vi "Write Cell T2.vi"(8 "error in (no error)":errorcluster, 10 "T2":dbl, 11 "cPAS Data in":refnum<class "cPAS Data.lvclass">) -> (0 "error out":errorcluster, 3 "cPAS Data out":refnum<class "cPAS Data.lvclass">)   [LabVIEW 2015, in "cPAS Data.lvclass"]
uses:
  cPAS Data.lvclass
  cPAS Cell Data/cPAS Cell Data.lvclass
  Reusable/PAS/Data/Main/Read CellData.vi
  Reusable/PAS/Data/Main/Read Current Cell.vi
  Reusable/PAS/Data/Main/Write CellData.vi
  Reusable/PAS/Data/Cell/PAS Cell Data.lvclass
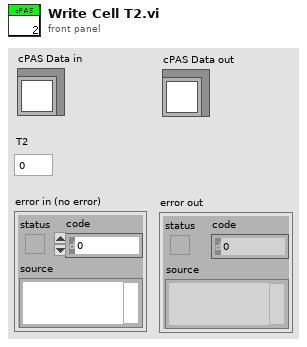
[diagram p1: front panel]
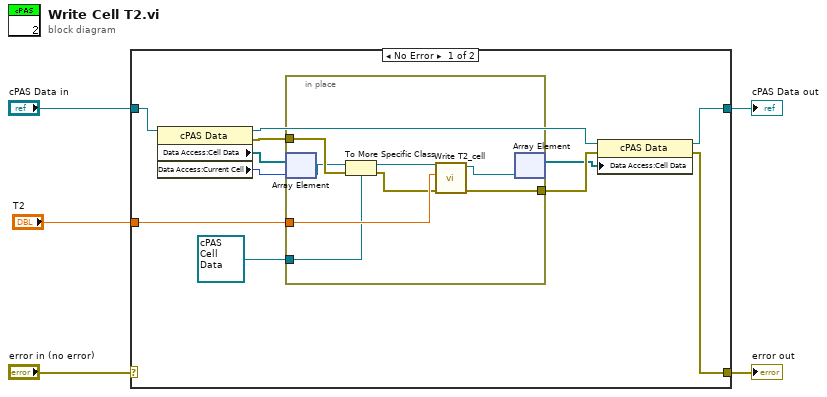
[diagram p0: block diagram]
diagram:
  n1 = case shown="No Error" "error in (no error)" {
    selector: "error in (no error)" -> [_ w26]
    tunnel: [w11 w26] -> w4
    tunnel: [w12 w25] -> w2
    tunnel: "cPAS Data in" -> [w16 w25]
    tunnel: "T2" -> [w15 _]
    frame No Error {
      n2 = property class="cPAS Data"(reference=w16) -> (reference out=w14:refnum<class "cPAS Data.lvclass">, error out=w10:errorcluster, "Data Access:Cell Data"=w9:refnum<class "PAS Cell Data.lvclass">[], "Data Access:Current Cell"=w8:i32)  [unwired: 1 in]
      n3 = in-place {
        in-place-border: w15 -> [w24]
        in-place-border: [w23] -> w13
        in-place-border: w10 -> [w21]
        in-place-border: refnum<class "cPAS Cell Data.lvclass"> refnum ("cPAS Cell in") -> [w18]
        n4 = in-place-array #1(w9, w8) -> (w17:refnum<class "PAS Cell Data.lvclass">)
        n5 = To More Specific Class(target class=w18, reference=w17, error in=w21) -> (specific class reference=w22:refnum<class "cPAS Cell Data.lvclass">, error out=w20:errorcluster)
        n6 = call "Write T2_cell.vi"("error in (no error)"=w20, "T2"=w24, "cPAS Cell in"=w22) -> ("error out"=w23:errorcluster, "cPAS Cell out"=w19:refnum<class "cPAS Cell Data.lvclass">)  [unwired: 7 in]
        n7 = in-place-array #1(w19) -> (w6:refnum<class "PAS Cell Data.lvclass">[])  [unwired: 1 out]
      }
      n8 = property class="cPAS Data"(reference=w14, error in=w13, "Data Access:Cell Data"=w6) -> (reference out=w12:refnum<class "cPAS Data.lvclass">, error out=w11:errorcluster)
    }
    frame Error {
    }
  }
  "error out" <- w4
  "cPAS Data out" <- w2
